vi "ziSetValueDemod.vi"(5 "Order (2)":i32=1 min=1, 6 "Rate (200Hz)":dbl=200.0, 7 "Time Constant (1ms)":dbl=0.001, 8 "error in":errorcluster, 9 "Signal Input Select (0)":i32, 10 "Demodulator # (0)":i32, 11 "handle in":T1 {"Handle" format="0x%08x"; "Conn" format="0x%08x"}) -> (0 "error out":errorcluster, 3 "handle out":T1 {"Handle" format="0x%08x"; "Conn" format="0x%08x"})   [LabVIEW 2009, in "Zurich Instruments LabOne.lvlib"]
doc: "Helper vi to comfortably configure a Demodulator. This vi brings a demodulator into a defined state by executing a number of setValueDouble calls."
uses:
  <instrlib>/Zurich Instruments LabOne/Zurich Instruments LabOne.lvlib
  <instrlib>/Zurich Instruments LabOne/Public/ziTypeHandle.ctl
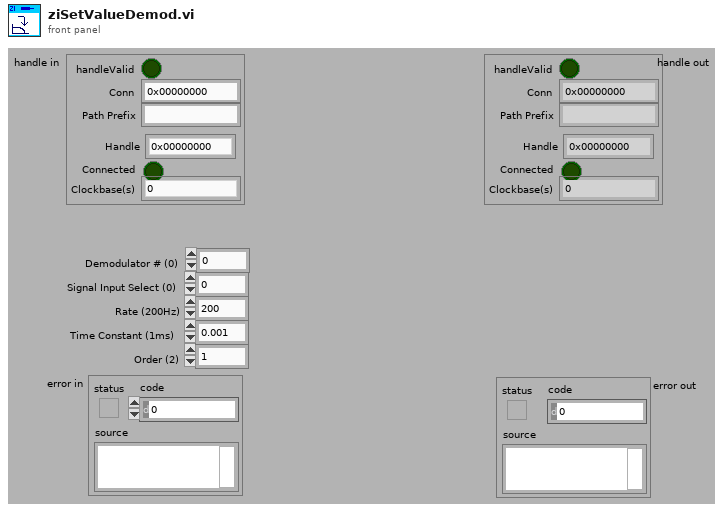
[diagram p1: front panel]
types:
  T1 = typedef "Zurich Instruments LabOne.lvlib/ziTypeHandle.ctl" = cluster{"handleValid":bool, "Conn":u64, "Path Prefix":string, "Handle":u64, "Connected":bool, "Clockbase(s)":dbl}
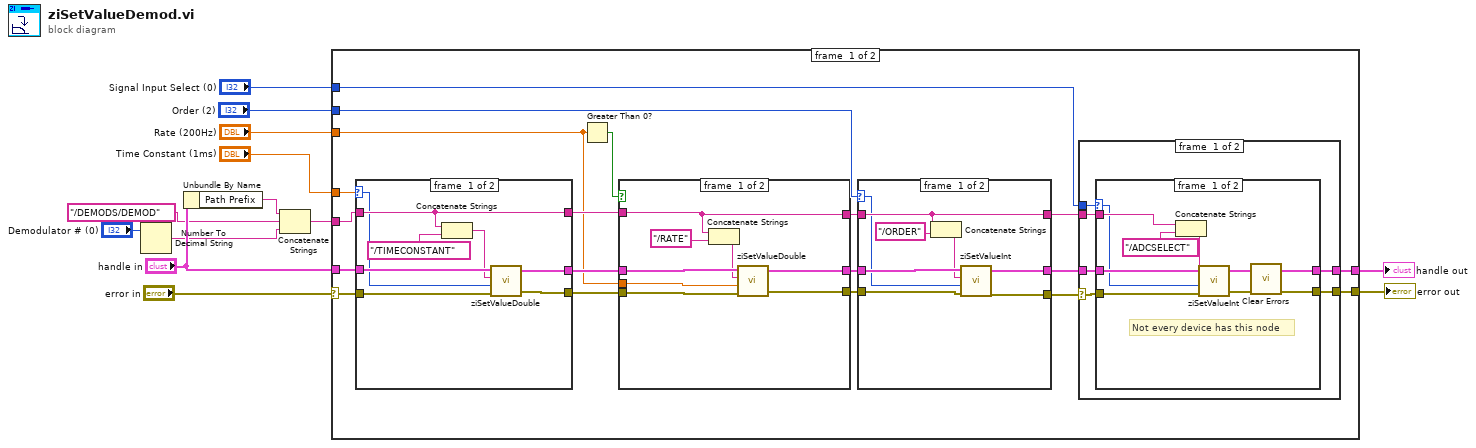
[diagram p0: block diagram]
diagram:
  n1 = Number To Decimal String(number="Demodulator # (0)") -> (decimal integer string=w4:string)  [unwired: 1 out]
  n2 = Unbundle By Name("handle in") -> ("Path Prefix"=w6:string)
  n3 = Concatenate Strings(w6, "/DEMODS/DEMOD", w4) -> (w3:string)
  n4 = case shown="No Error" "error in" {
    selector: "error in" -> [w14 w86]
    tunnel: "Time Constant (1ms)" -> [w32 _]
    tunnel: "Order (2)" -> [w31 _]
    tunnel: "Signal Input Select (0)" -> [w30 _]
    tunnel: [w26 w85] -> w10
    tunnel: [w23 w86] -> w9
    tunnel: "handle in" -> [w22 w85]
    tunnel: w3 -> [w18 _]
    tunnel: "Rate (200Hz)" -> [w16 _]
    frame #0 {
      n5 = case shown="Default" w32 {
        selector: w32 -> [w74 _]
        tunnel: w22 -> [w81 w84]
        tunnel: [w80 w84] -> w29
        tunnel: [w79 w83] -> w24
        tunnel: w14 -> [w78 w83]
        tunnel: w18 -> [w77 w82]
        tunnel: [w77 w82] -> w21
        frame #0 {
          n6 = Concatenate Strings(w77, "/TIMECONSTANT") -> (w75:string)
          n7 = call <instrlib>:"ziSetValueDouble.vi"("Error In"=w78, "Value"=w74, "Path"=w75, "Handle In"=w81) -> ("Error Out"=w79:errorcluster, "Handle Out"=w80:T1)  [unwired: 1 in]
        }
        frame #1 {
        }
      }
      n8 = Greater Than 0?(x=w16) -> (x > 0?=w17:bool)
      n9 = case shown="True" w17 {
        tunnel: w29 -> [w70 w73]
        tunnel: [w69 w73] -> w28
        tunnel: [w68 w72] -> w25
        tunnel: w24 -> [w67 w72]
        tunnel: w21 -> [w64 w71]
        tunnel: [w64 w71] -> w20
        tunnel: w16 -> [w63 _]
        frame #0 {
          n10 = Concatenate Strings(w64, "/RATE") -> (w65:string)
          n11 = call <instrlib>:"ziSetValueDouble.vi"("Error In"=w67, "Value"=w63, "Path"=w65, "Handle In"=w70) -> ("Error Out"=w68:errorcluster, "Handle Out"=w69:T1)  [unwired: 1 out]
        }
        frame #1 {
        }
      }
      n12 = case shown="Default" w31 {
        selector: w31 -> [w52 _]
        tunnel: w28 -> [w59 w62]
        tunnel: [w58 w62] -> w27
        tunnel: [w57 w61] -> w15
        tunnel: w25 -> [w56 w61]
        tunnel: w20 -> [w53 w60]
        tunnel: [w53 w60] -> w19
        frame #0 {
          n13 = Concatenate Strings(w53, "/ORDER") -> (w54:string)
          n14 = call <instrlib>:"ziSetValueInt.vi"("Error in"=w56, "Value"=w52, "Path"=w54, "Handle in"=w59) -> ("Error out"=w57:errorcluster, "Handle out"=w58:T1)  [unwired: 1 out]
        }
        frame #1 {
        }
      }
      n15 = case shown="No Error" w15 {
        selector: w15 -> [w33 w50]
        tunnel: w30 -> [w38 _]
        tunnel: w27 -> [w37 w51]
        tunnel: [w36 w51] -> w26
        tunnel: [w35 w50] -> w23
        tunnel: w19 -> [w34 _]
        frame #0 {
          n16 = case shown="Default" w38 {
            selector: w38 -> [w40 _]
            tunnel: w37 -> [w47 w49]
            tunnel: [w46 w49] -> w36
            tunnel: w33 -> [w45 w48]
            tunnel: [w39 w48] -> w35
            tunnel: w34 -> [w43 _]
            frame #0 {
              # "Not every device has this node"
              n17 = Concatenate Strings(w43, "/ADCSELECT") -> (w42:string)
              n18 = call <instrlib>:"ziSetValueInt.vi"("Error in"=w45, "Value"=w40, "Path"=w42, "Handle in"=w47) -> ("Error out"=w44:errorcluster, "Handle out"=w46:T1)  [unwired: 1 out]
              n19 = call <vilib>:"Clear Errors.vi"("error in (no error)"=w44) -> ("error out"=w39:errorcluster)  [unwired: 6 in]
            }
            frame #1 {
            }
          }
        }
        frame #1 {
        }
      }
    }
    frame #1 {
    }
  }
  "handle out" <- w10
  "error out" <- w9
